vi "config Spark Max.vi"(11 "motor\ndefaults":T1 {"MOTOR SELECT" items=["REV NEO"=5676, "REV NEO 550"=11000, "VEX Falcon"=6380, "WC Kraken"=6000]}) -> (0 "error out":errorcluster, 3 "MotorControlDevRef":T5)   [LabVIEW 2023]
uses:
  <vilib>/Rock Robotics/WPI/MotorControl/WPI_MotorControlDeviceRef.ctl
  <vilib>/Rock Robotics/WPI/MotorControl/WPI_MotorControlType.ctl
  <vilib>/Rock Robotics/SystemInterfaces/DIO/FPGA_DIOPWMChannel.ctl
  <vilib>/Rock Robotics/WPI/PWM/WPI_PWMDeadband.ctl
  <vilib>/Rock Robotics/SystemInterfaces/DIO/FPGA_DIOChannel.ctl
  ctrl defs/ctrl swerve motor.ctl
  ctrl defs/ctrl MOTOR SELECT.ctl
  <vilib>/Rock Robotics/WPI/ThirdParty/REV Robotics/REVLib/Typedef/Spark MAX Idle Mode.ctl
  ctrl defs/ctrl Spark MAX current limiting.ctl
  <vilib>/Rock Robotics/WPI/ThirdParty/REV Robotics/REVLib/Typedef/Spark MAX Motor Type.ctl
  <vilib>/Rock Robotics/WPI/ThirdParty/REV Robotics/REVLib/Typedef/Spark MAX Limit Switch Polarity.ctl
  <vilib>/Rock Robotics/WPI/ThirdParty/REV Robotics/REVLib/Typedef/Spark MAX Limit Direction.ctl
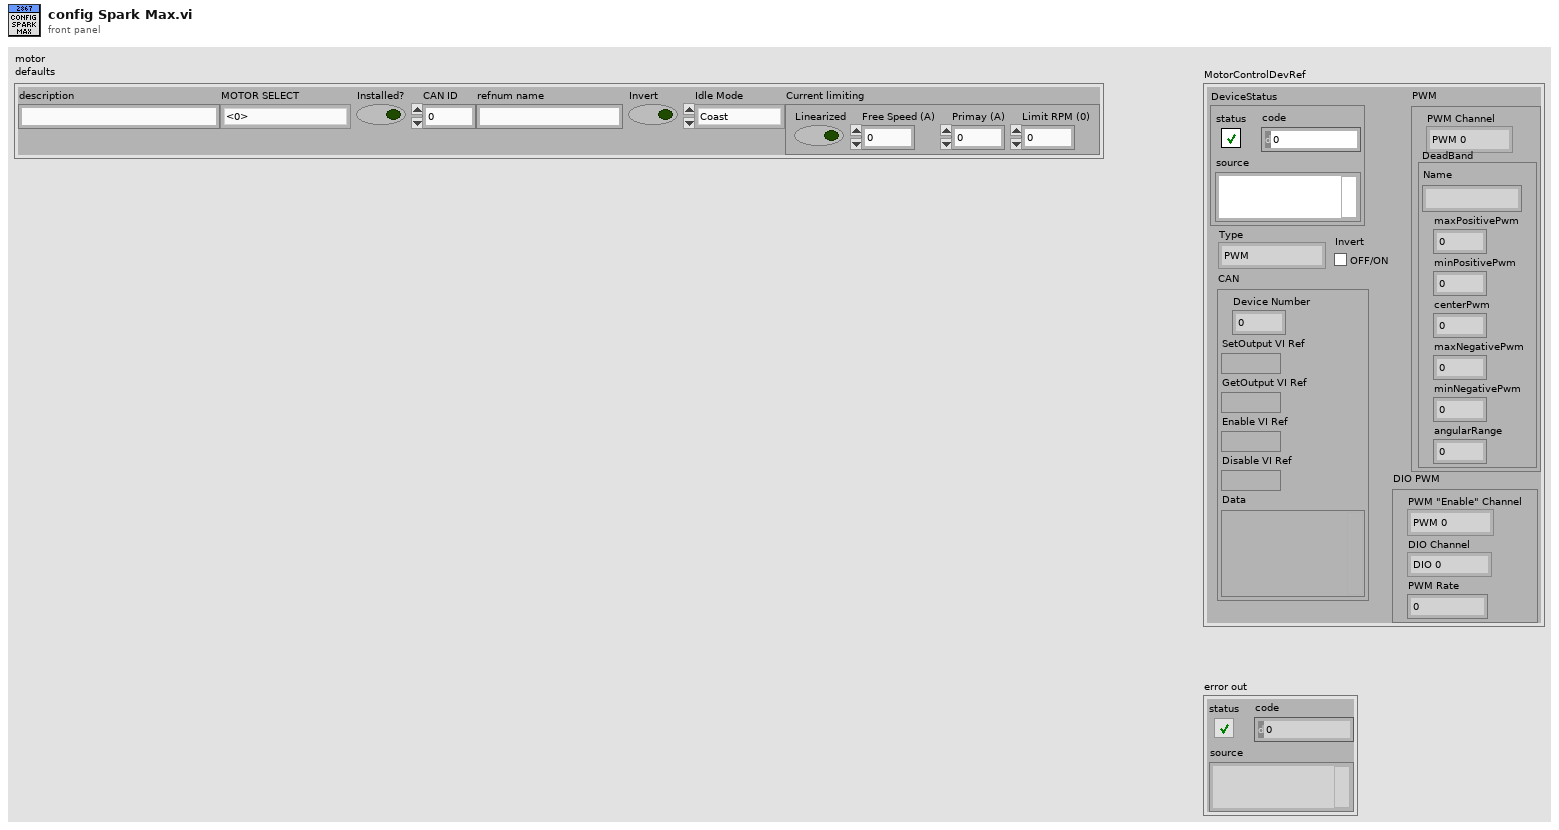
[diagram p1: front panel]
types:
  T1 = typedef "ctrl swerve motor.ctl" = cluster{"description":string, "MOTOR SELECT":T2, "Installed?":bool, "CAN ID":u8, "refnum name":string, "Invert":bool, "Idle Mode":T3, "Current limiting":T4}
  T2 = typedef "ctrl MOTOR SELECT.ctl" = i16
  T3 = typedef "Spark MAX Idle Mode.ctl" = enum16{"Coast", "Brake"}
  T4 = typedef "ctrl Spark MAX current limiting.ctl" = cluster{"Linearized":bool, "Free Speed (A)":dbl, "Primay (A)":dbl, "Limit RPM (0)":u32}
  T5 = typedef "WPI_MotorControlDeviceRef.ctl" = cluster{"DeviceStatus":errorcluster, "Type":T6, "PWM":cluster{"PWM Channel":T7, "DeadBand":T8}, "CAN":cluster{"Device Number":u8, "SetOutput VI Ref":variant, "GetOutput VI Ref":variant, "Enable VI Ref":variant, "Disable VI Ref":variant, "Data":variant}, "Invert":bool, "DIO PWM":cluster{"PWM \"Enable\" Channel":T7, "DIOChannel":T9, "PWM Rate":dbl}}
  T6 = typedef "WPI_MotorControlType.ctl" = enum16{"PWM", "CAN", "DIO PWM"}
  T7 = typedef "FPGA_DIOPWMChannel.ctl" = enum8{"PWM 0", "PWM 1", "PWM 2", "PWM 3", "PWM 4", "PWM 5", "PWM 6", "PWM 7", "PWM 8", "PWM 9", "PWM MXP 0", "PWM MXP 1", "PWM MXP 2", "PWM MXP 3", "PWM MXP 4", "PWM MXP 5", "PWM MXP 6", "PWM MXP 7", "PWM MXP 8", "PWM MXP 9", "Invalid"}
  T8 = typedef "WPI_PWMDeadband.ctl" = cluster{"Name":string, "maxPositivePwm":i32, "minPositivePwm":i32, "centerPwm":i32, "maxNegativePwm":i32, "minNegativePwm":i32, "angularRange":u16}
  T9 = typedef "FPGA_DIOChannel.ctl" = enum8{"DIO 0", "DIO 1", "DIO 2", "DIO 3", "DIO 4", "DIO 5", "DIO 6", "DIO 7", "DIO 8", "DIO 9", "DIO MXP 0", "DIO MXP 1", "DIO MXP 2", "DIO MXP 3", "DIO MXP 4", "DIO MXP 5", "DIO MXP 6", "DIO MXP 7", "DIO MXP 8", "DIO MXP 9", "DIO MXP 10", "DIO MXP 11", "DIO MXP 12", "DIO MXP 13", "DIO MXP 14", "DIO MXP 15", "SPI Port CS1", "SPI Port CS2", "SPI Port CS3", "SPI Port MISO", "SPI Port MOSI", "Invalid"}
  T10 = typedef "Spark MAX Motor Type.ctl" = enum16{"Brushed", "Brushless"}
  T11 = typedef "Spark MAX Limit Direction.ctl" = enum16{"Forward Limit", "Reverse Limit"}
  T12 = typedef "Spark MAX Limit Switch Polarity.ctl" = enum16{"Normally Open", "Normally Closed"}
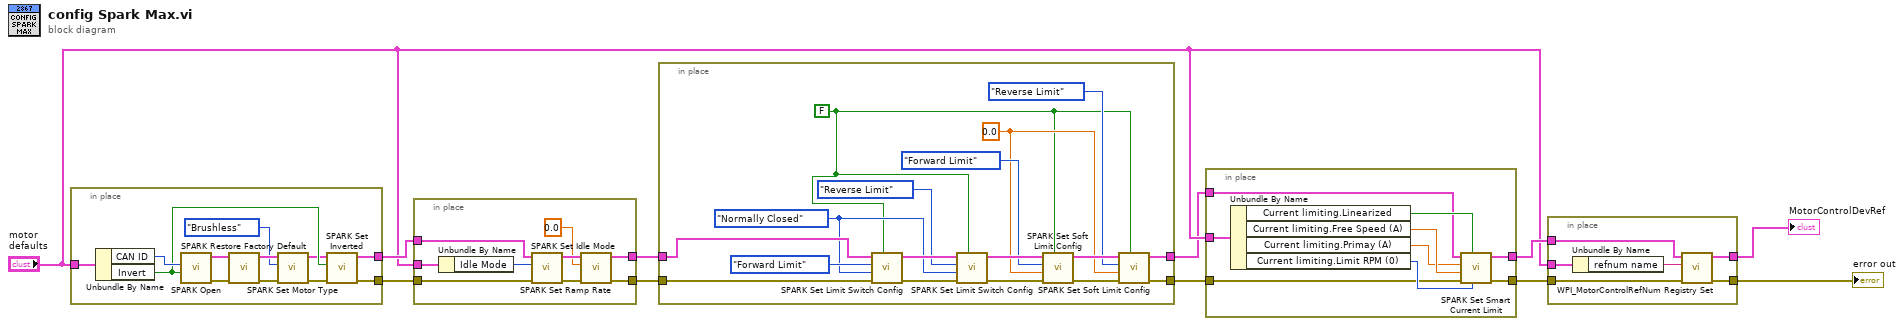
[diagram p0: block diagram]
diagram:
  n1 = in-place {
    in-place-border: [w21] -> w7
    in-place-border: [w20] -> w6
    in-place-border: "motor\ndefaults" -> [w16]
    n2 = Unbundle By Name(w16) -> ("CAN ID"=w23:u8, "Invert"=w22:bool)
    n3 = call <vilib>:"SPARK Open.vi"("Invert"=w22, "Device Number"=w23) -> ("error out"=w17:errorcluster, "MotorControlDeviceRef"=w18:T5)  [unwired: 8 in]
    n4 = call <vilib>:"SPARK Restore Factory Default.vi"("error in"=w17, "MotorControlDeviceRef"=w18) -> ("error out"=w14:errorcluster, "MotorControlDeviceRef"=w19:T5)  [unwired: 8 in]
    n5 = call <vilib>:"SPARK Set Motor Type.vi"("error in (no error)"=w14, "Motor Type"=Spark_MAX_Motor_Type."Brushless", "MotorControlDevRef"=w19) -> ("error out"=w13:errorcluster, "MotorControlDeviceRef"=w15:T5)  [unwired: 7 in]
    n6 = call <vilib>:"SPARK Set Inverted.vi"("error in (no error)"=w13, "Inverted (F)"=w22, "MotorControlDeviceRef in"=w15) -> ("error out"=w21:errorcluster, "MotorControlDeviceRef out"=w20:T5)  [unwired: 7 in]
  }
  n7 = in-place {
    in-place-border: w7 -> [w32]
    in-place-border: w6 -> [w31]
    in-place-border: [w27] -> w5
    in-place-border: [w25] -> w2
    in-place-border: "motor\ndefaults" -> [w28]
    n8 = Unbundle By Name(w28) -> ("Idle Mode"=w29:T3)
    n9 = call <vilib>:"SPARK Set Idle Mode.vi"("error in (no error)"=w32, "Idle Mode"=w29, "MotorControlDeviceRef in"=w31) -> ("error out"=w26:errorcluster, "MotorControlDeviceRef out"=w30:T5)  [unwired: 7 in]
    n10 = call <vilib>:"SPARK Set Ramp Rate.vi"("error in (no error)"=w26, "Seconds from neutral to full (0)"=sgl 0.0, "MotorControlDeviceRef in"=w30) -> ("error out"=w25:errorcluster, "MotorControlDeviceRef"=w27:T5)  [unwired: 7 in]
  }
  n11 = in-place {
    in-place-border: w5 -> [w49]
    in-place-border: [w39] -> w3
    in-place-border: w2 -> [w43]
    in-place-border: [w33] -> w1
    w37 = 0.0 ("Soft Limit (0)")
    w44 = Spark_MAX_Limit_Switch_Polarity."Normally Closed" ("Polarity (Normally Open)")
    w36 = FALSE ("Enabled? (T)")
    n12 = call <vilib>:"SPARK Set Limit Switch Config.vi"("Enabled? (T)"=w36, "error in (no error)"=w43, "Polarity (Normally Open)"=w44, "Limit Switch"=Spark_MAX_Limit_Direction."Forward Limit", "MotorControlDeviceRef in"=w49) -> ("error out"=w42:errorcluster, "MotorControlDeviceRef out"=w48:T5)  [unwired: 5 in]
    n13 = call <vilib>:"SPARK Set Limit Switch Config.vi"("Enabled? (T)"=w36, "error in (no error)"=w42, "Polarity (Normally Open)"=w44, "Limit Switch"=Spark_MAX_Limit_Direction."Reverse Limit", "MotorControlDeviceRef in"=w48) -> ("error out"=w35:errorcluster, "MotorControlDeviceRef out"=w46:T5)  [unwired: 5 in]
    n14 = call <vilib>:"SPARK Set Soft Limit Config.vi"("Enabled? (T)"=w36, "error in (no error)"=w35, "Soft Limit (0)"=w37, "Soft Limit Switch"=Spark_MAX_Limit_Direction."Forward Limit", "MotorControlDeviceRef in"=w46) -> ("error out"=w34:errorcluster, "MotorControlDeviceRef out"=w41:T5)  [unwired: 5 in]
    n15 = call <vilib>:"SPARK Set Soft Limit Config.vi"("Enabled? (T)"=w36, "error in (no error)"=w34, "Soft Limit (0)"=w37, "Soft Limit Switch"=Spark_MAX_Limit_Direction."Reverse Limit", "MotorControlDeviceRef in"=w41) -> ("error out"=w33:errorcluster, "MotorControlDeviceRef out"=w39:T5)  [unwired: 5 in]
  }
  n16 = in-place {
    in-place-border: [w58] -> w10
    in-place-border: [w53] -> w8
    in-place-border: w3 -> [w52]
    in-place-border: w1 -> [w51]
    in-place-border: "motor\ndefaults" -> [w50]
    n17 = Unbundle By Name(w50) -> ("Current limiting.Linearized"=w54:bool, "Current limiting.Free Speed (A)"=w56:dbl, "Current limiting.Primay (A)"=w55:dbl, "Current limiting.Limit RPM (0)"=w57:u32)
    n18 = call <vilib>:"SPARK Set Smart Current Limit.vi"("Linear Limit RPM (0)"=w57, "Linearized Limit Enabled (F)"=w54, "error in (no error)"=w51, "Free Speed Current Limit (20A)"=w56, "Primay Current Limit (80A)"=w55, "MotorControlDeviceRef in"=w52) -> ("error out"=w58:errorcluster, "MotorControlDeviceRef out"=w53:T5)  [unwired: 4 in]
  }
  n19 = in-place {
    in-place-border: [w64] -> w11
    in-place-border: w10 -> [w63]
    in-place-border: [w62] -> w9
    in-place-border: w8 -> [w61]
    in-place-border: "motor\ndefaults" -> [w59]
    n20 = Unbundle By Name(w59) -> ("refnum name"=w60:string)
    n21 = call <vilib>:"WPI_MotorControlRefNum Registry Set.vi"("error in (no error)"=w63, "refnum name"=w60, "MotorControlDevRef"=w61) -> ("error out"=w64:errorcluster, "MotorControlDevRef"=w62:T5)  [unwired: 7 in]
  }
  "error out" <- w11
  "MotorControlDevRef" <- w9
